vi "main_lidar-to-grid-map.vi"() -> ()   [LabVIEW 2019]
uses:
  Ctrl/cmd_common.ctl
  <vilib>/Utility/file.llb/Read Delimited Spreadsheet (DBL).vi
panel:
  in  "탭 컨트롤":enum32{"페이지 1", "페이지 2"}(tab)
  in  "xy_resolution":dbl=0.02
  in  "EXTEND_AREA":dbl=1.0
  out "배열":dbl[](array[numeric])
  out "i":i32
  out "웨이브폼 그래프":dbl[](graph)
  out "Raw map":cluster{"X":dbl, "Y":dbl}[](graph)
  # "Lidar to Gridmap"
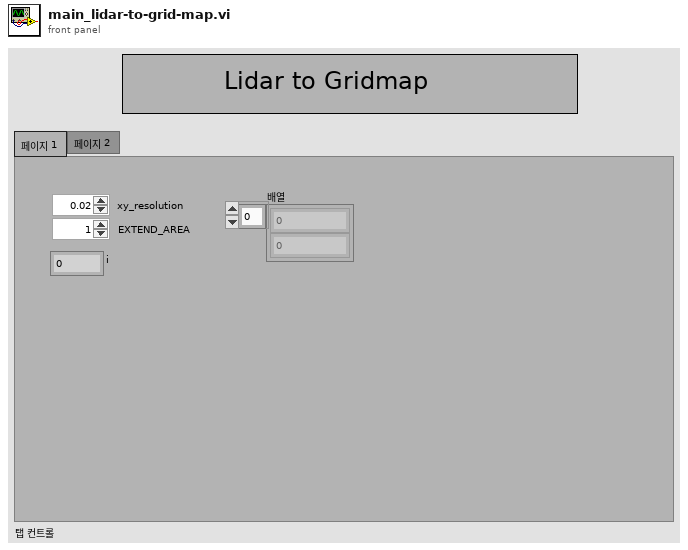
[diagram p1: front panel]
types:
  T1 = typedef "cmd_common.ctl" = enum16{"read", "write"}
  T2 = typedef "NI_Matrix.lvlib/RealMatrix.ctl" = dbl[][]
  T3 = cluster{"resolution":dbl, "EXTEND_AREA":dbl, "MAX_RANGE":dbl, "NP":u32, "NTh":u32, "Q":T2, "R":T2, "Q_sim":T2, "R_sim":T2, "rf_id":cluster{"x":dbl, "y":dbl}[]}
  T4 = cluster{"ox":T2, "oy":T2, "occupancy map":T2, "x_true":T2, "u":T2, "z":T2, "PEst":T2, "min x":dbl, "min y":dbl, "max x":dbl, "max y":dbl, "yw":i32, "xw":i32}
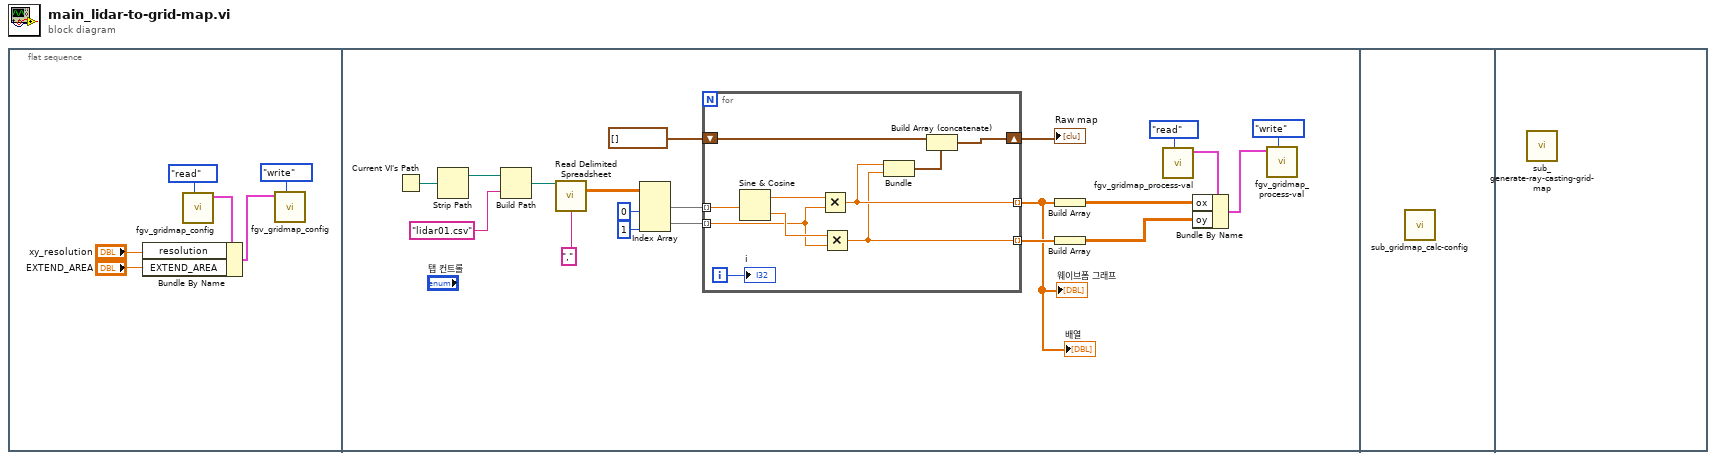
[diagram p0: block diagram]
diagram:
  n1 = flat-sequence {
    frame #0 {
      n2 = call "fgv_gridmap_config.vi"("cmd"=cmd_common."read") -> ("pf-val out"=w4:T3)  [unwired: 10 in]
      n3 = Bundle By Name(cluster=w4, "resolution"="xy_resolution", "EXTEND_AREA"="EXTEND_AREA") -> (w2:T3)
      n4 = call "fgv_gridmap_config.vi"("cmd"=cmd_common."write", "pf-val"=w2) -> ()  [unwired: 9 in, 1 out]
    }
    frame #1 {
      n5 = Current VI's Path() -> (path=w18:path)
      n6 = Strip Path(path=w18) -> (stripped path=w17:path)  [unwired: 1 out]
      n7 = Build Path(base path=w17, name or relative path="lidar01.csv" ("이름 또는 상대 경로")) -> (appended path=w15:path)
      n8 = call-poly <vilib>:"Read Delimited Spreadsheet.vi"("file path (dialog if empty)"=w15, "delimiter (\\t)"="," ("delimiter (\\t)")) -> ("all rows"=w25:dbl[][])  [unwired: 8 in, 5 out]
      n9 = Index Array(array=w25, index (col) #1=0 ("비활성화된 인덱스 (열)"), index (col) #2=1 ("인덱스 (열)")) -> (element #1=w22:dbl[], element #2=w20:dbl[])  [unwired: 2 in]
      n10 = for {
        tunnel: w22 -> [w36] mode=indexing
        shift-right: [w30] -> w19
        shift-left: cluster{"x":dbl, "y":dbl}[] [] -> [w35]
        tunnel: w20 -> [w32] mode=indexing
        tunnel: [w28] -> w7 mode=indexing
        tunnel: [w27] -> w12 mode=indexing
        i -> [w29]
        n11 = Sine & Cosine(0:w36) -> (1:w34:dbl, 2:w33:dbl)
        n12 = Multiply(x=w34, y=w32) -> (x*y=w28:dbl)
        n13 = Multiply(x=w33, y=w32) -> (x*y=w27:dbl)
        n14 = Bundle(w28, w27) -> (w31:cluster{dbl, dbl})  [unwired: 1 in]
        n15 = Build Array (concatenate)(w35, w31) -> (w30:cluster{"x":dbl, "y":dbl}[])
        "i" <- w29
      }
      "Raw map" <- w19
      "웨이브폼 그래프" <- w7
      "배열" <- w7
      n16 = Build Array(w7) -> (w10:T2)
      n17 = Build Array(w12) -> (w8:T2)
      n18 = call "fgv_gridmap_process-val.vi"("cmd"=cmd_common."read") -> ("p-val  2"=w11:T4)  [unwired: 10 in]
      n19 = Bundle By Name(cluster=w11, "ox"=w10, "oy"=w8) -> (w9:T4)
      n20 = call "fgv_gridmap_process-val.vi"("cmd"=cmd_common."write", "p-val"=w9) -> ()  [unwired: 9 in, 1 out]
    }
    frame #2 {
      n21 = call "sub_gridmap_calc-config.vi"() -> ()  [unwired: 12 in]
    }
    frame #3 {
      n22 = call "sub_generate-ray-casting-grid-map.vi"() -> ()  [unwired: 12 in]
    }
  }
